vi "Create and Configure Signal Configuration.vi"(8 "error in":errorcluster, 11 "Measurement configuration":T1={"Full scale range"=3.16, "Maximum harmonic"=5, "Analog source resource name"="", "Frequency start"=100.0, "Frequency stop"=20000.0, "Frequency steps"=50, "Frequency spacing"="", "Amplitude"=1.0, "DC Offset"=0.0, "Measurement duration"=0.001, "Measurement cycles"=10, "Settling time"=0.0, "Settling cycles"=0, "Protocol capture resource name"="", "Data line"=0, "Channel"=0, "Sample rate"=12288000.0, "Frame sync edge for channel 0"=1, "Channel count per frame"=2, "Channel length"=32, "Bit depth"=24, "Channel 0 offset"=1, "Endianness"=0, "Data justification"=0, "Frame length"=64, "Frame sync pulse width"=32, "Bit clock edge sync"=1} {"Settling cycles" min=0 max=5 step=1 format="%.3f"}) -> (0 "error out":errorcluster, 1 "duration":dbl, 3 "signal configuration":refnum<class "SV Discrete Sweep.lvclass">)   [LabVIEW 2021, in "Frequency Response_Audio ADC.lvlib"]
uses:
  Frequency Response_Audio ADC.lvlib
  Measurement Configuration.ctl
  <vilib>/addons/_NISVFA/_Generation/Signal Generation/SV Discrete Sweep/SV Discrete Sweep.lvclass
  C:/Program Files/National Instruments/LabVIEW 2021/vi.lib/addons/_NISVFA/_Generation/Signal Generation/SV Signal/SV Signal.lvclass
  C:/Program Files/National Instruments/LabVIEW 2021/vi.lib/addons/_NISVFA/_Generation/Signal Generation/SV Function/SV Function.lvclass
  <vilib>/addons/_NISVFA/_Generation/Signal Generation/SV Signal/SV Signal.lvclass/SV Signal.ctl
  <vilib>/addons/_NISVFA/_Generation/Signal Generation/SV Signal/Write Leading Synchronization Pulse Enable.vi
  <vilib>/addons/_NISVFA/_Generation/Signal Generation/SV Signal/Read Total Samples.vi
  <vilib>/addons/_NISVFA/_Generation/Signal Generation/SV Signal/Calculate Number of Remaining Samples.vi
  <vilib>/addons/_NISVFA/_Generation/Signal Generation/SV Discrete Sweep/Configure Frequency Sweep at Constant Amplitude.vi
  <vilib>/addons/_NISVFA/_Generation/Signal Generation/SV Signal/Write Ramp Parameters.vi
  <vilib>/addons/_NISVFA/_Generation/Signal Generation/SV Signal/Write DC Offset.vi
  <vilib>/addons/_NISVFA/_Generation/Signal Generation/SV Signal/Write Measurement Duration.vi
  <vilib>/addons/_NISVFA/_Generation/Signal Generation/SV Function/Write Measurement Cycles.vi
  <vilib>/addons/_NISVFA/_Generation/Signal Generation/SV Signal/Write Pre-Measurement Settling Duration.vi
  <vilib>/addons/_NISVFA/_Generation/Signal Generation/SV Function/Write Pre-Measurement Settling Cycles.vi
  <vilib>/addons/_NISVFA/_Generation/Signal Generation/SV Signal/Read Generation State.vi
  <vilib>/addons/_NISVFA/_Generation/Signal Generation/SV Signal/Read System Timing Model.vi
  <vilib>/addons/_NISVFA/_Generation/Signal Generation/SV Signal/Read Sample Rate.vi
  <vilib>/addons/_NISVFA/_Generation/Signal Generation/SV Signal/SV Signal.lvclass
  shared/Audio ADC Shared.lvlib
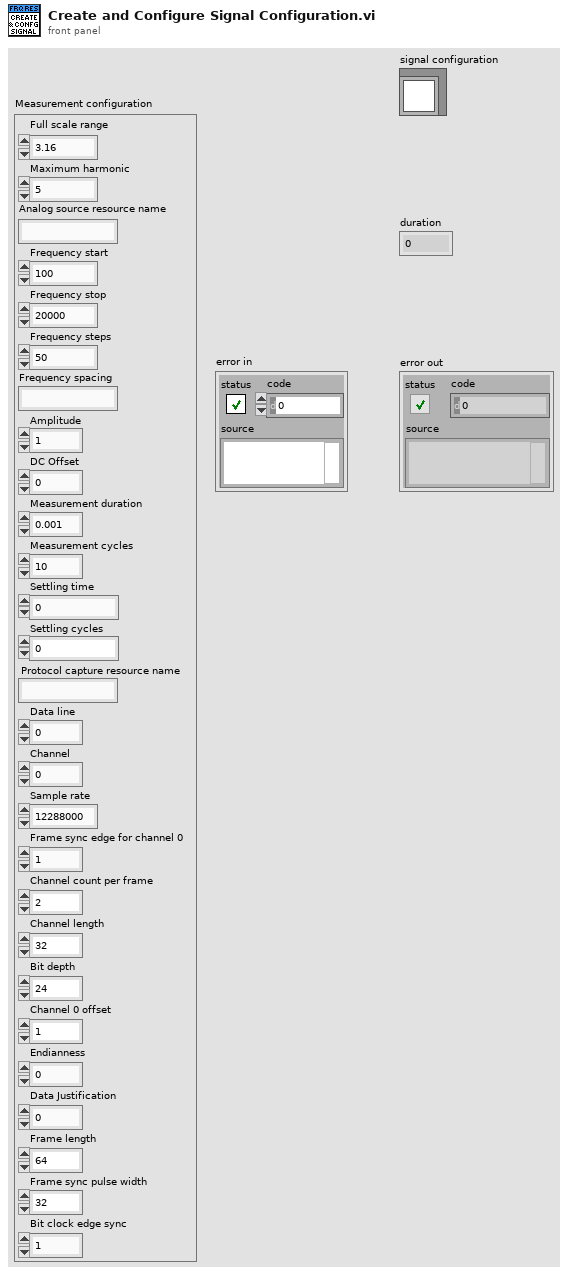
[diagram p1: front panel]
types:
  T1 = typedef "Frequency Response_Audio ADC.lvlib/Measurement Configuration.ctl" = cluster{"Full scale range":dbl, "Maximum harmonic":i32, "Analog source resource name":string, "Frequency start":dbl, "Frequency stop":dbl, "Frequency steps":i32, "Frequency spacing":string, "Amplitude":dbl, "DC Offset":dbl, "Measurement duration":dbl, "Measurement cycles":i32, "Settling time":dbl, "Settling cycles":i32, "Protocol capture resource name":string, "Data line":u32, "Channel":u32, "Sample rate":dbl, "Frame sync edge for channel 0":u32, "Channel count per frame":u32, "Channel length":u32, "Bit depth":u32, "Channel 0 offset":u32, "Endianness":u32, "Data justification":u32, "Frame length":u32, "Frame sync pulse width":u32, "Bit clock edge sync":u32}
  T2 = cluster{"profile":enum16{"Linear", "Half cosine"}, "durations [s]":cluster{"ramp-up":dbl, "transition":dbl, "ramp-down":dbl}}
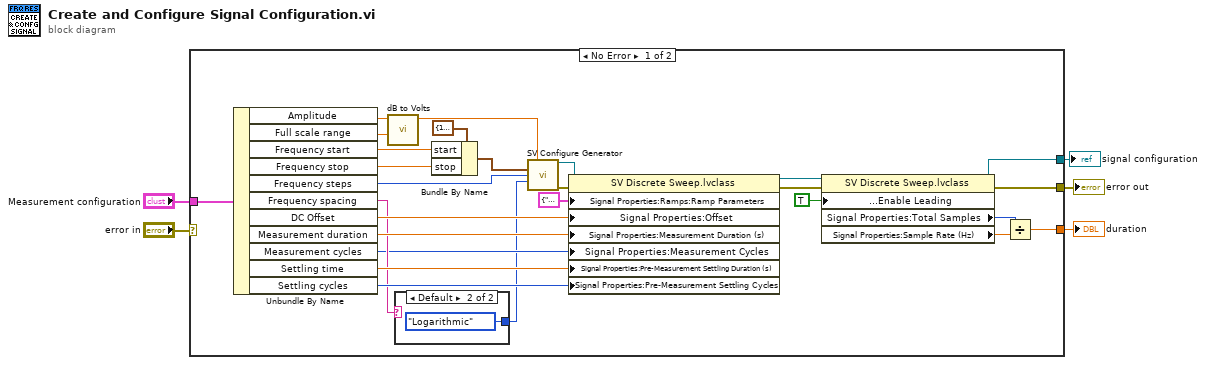
[diagram p0: block diagram]
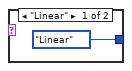
[diagram p2: hidden frame]
diagram:
  n1 = case shown="No Error" "error in" {
    selector: "error in" -> [_ w35]
    tunnel: "Measurement configuration" -> [w32 _]
    tunnel: [w11 w35] -> w3
    tunnel: [w10 _] -> w1
    tunnel: [w9 _] -> w2
    frame No Error {
      n2 = Unbundle By Name(w32) -> ("Amplitude"=w30:dbl, "Full scale range"=w31:dbl, "Frequency start"=w27:dbl, "Frequency stop"=w26:dbl, "Frequency steps"=w24:i32, "Frequency spacing"=w8:string, "DC Offset"=w20:dbl, "Measurement duration"=w19:dbl, "Measurement cycles"=w7:i32, "Settling time"=w18:dbl, "Settling cycles"=w17:i32)
      n3 = call "dB to Volts.vi"("Full scale range"=w31, "Voltage(dB)"=w30) -> ("Voltage(volts)"=w29:dbl)  [unwired: 9 in]
      n4 = case shown="Default" w8 {
        tunnel: [enum16{"Linear", "Logarithmic"}."Linear" ("profile") enum16{"Linear", "Logarithmic"}."Logarithmic" ("profile")] -> w6
        frame "Linear" {
        }
        frame Default {
        }
      }
      n5 = Bundle By Name(cluster=cluster{"start":dbl, "stop":dbl} {"start"=10.0, "stop"=10000.0} ("frequency range [Hz]"), "start"=w27, "stop"=w26) -> (w25:cluster{"start":dbl, "stop":dbl})
      n6 = call-poly <vilib>:"SV Configure Generator.vi"("amplitude"=w29, "frequency range [Hz]"=w25, "number of steps"=w24, "profile"=w6) -> ("signal configuration"=w21:refnum<class "SV Discrete Sweep.lvclass">, "error out"=w22:errorcluster)  [unwired: 10 in]
      n7 = property class="SV Discrete Sweep.lvclass"(reference=w21, error in=w22, "Signal Properties:Ramps:Ramp Parameters"=T2 {"profile"=enum."Half cosine", "durations [s]"={"ramp-up"=0.01, "transition"=0.0, "ramp-down"=0.01}} ("Ramp Parameters"), "Signal Properties:Offset"=w20, "Signal Properties:Measurement Duration (s)"=w19, "Signal Properties:Measurement Cycles"=w7, "Signal Properties:Pre-Measurement Settling Duration (s)"=w18, "Signal Properties:Pre-Measurement Settling Cycles"=w17) -> (reference out=w15:refnum<class "SV Discrete Sweep.lvclass">, error out=w14:errorcluster)
      n8 = property on="Property Node" class="SV Discrete Sweep.lvclass"(reference=w15, error in=w14, "Signal Properties:Synchronization Pulses:Enable Leading"=TRUE ("Synchronization Pulses:Enable Leading")) -> (reference out=w10:refnum<class "SV Discrete Sweep.lvclass">, error out=w11:errorcluster, "Signal Properties:Total Samples"=w13:i32, "Signal Properties:Sample Rate (Hz)"=w12:dbl)
      n9 = Divide(x=w13, y=w12) -> (x/y=w9:dbl)
    }
    frame Error {
    }
  }
  "error out" <- w3
  "duration" <- w2
  "signal configuration" <- w1
